vi "CollectionStatus.vi"(8 "error in (no error)":errorcluster, 11 "controller in":refnum<k24>) -> (0 "error out":errorcluster, 1 "PointsCollected":i32, 2 "IsCollecting":bool, 3 "controller out":refnum<k24>, 4 "PointsAllocated":i32, 6 "PointsRetrieved":i32)   [LabVIEW 2016, in "Aerotech VIs.lvlib"]
uses:
  Aerotech VIs.lvlib
  C:/Program Files (x86)/Aerotech/A3200/LabVIEW/2010/Bin/Aerotech.A3200.dll
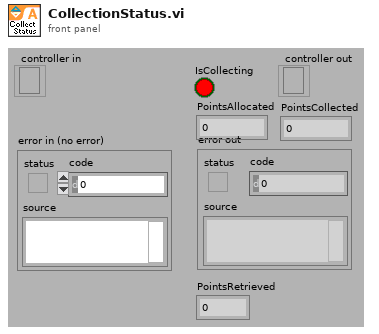
[diagram p1: front panel]
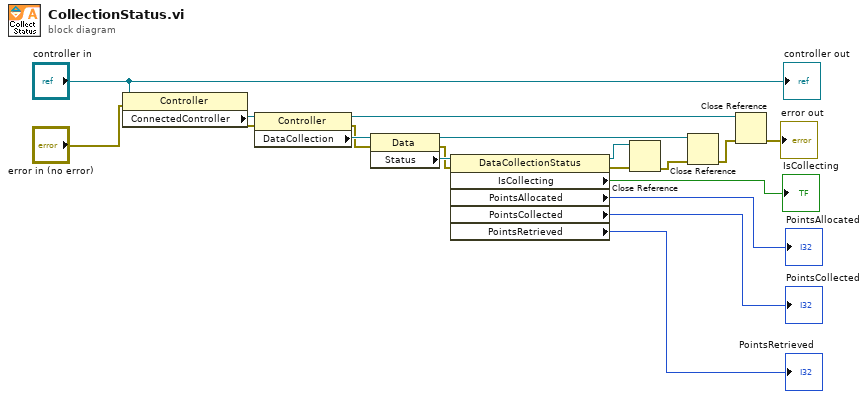
[diagram p0: block diagram]
diagram:
  n1 = property class="Controller"(reference="controller in", error in="error in (no error)") -> (error out=w17:errorcluster, "ConnectedController"=w18:refnum<k24>)  [unwired: 1 out]
  n2 = property class="Controller"(reference=w18, error in=w17) -> (reference out=w10:refnum<k24>, error out=w14:errorcluster, "DataCollection"=w16:refnum<k24>)
  n3 = property class="Data"(reference=w16, error in=w14) -> (reference out=w12:refnum<k24>, error out=w7:errorcluster, "Status"=w8:refnum<k24>)
  n4 = property class="DataCollectionStatus"(reference=w8, error in=w7) -> (reference out=w2:refnum<k24>, error out=w3:errorcluster, "IsCollecting"=→"IsCollecting":bool, "PointsAllocated"=→"PointsAllocated":i32, "PointsCollected"=→"PointsCollected":i32, "PointsRetrieved"=→"PointsRetrieved":i32)
  n5 = Close Reference(reference=w2, error in (no error)=w3) -> (error out=w13:errorcluster)
  n6 = Close Reference(reference=w12, error in (no error)=w13) -> (error out=w11:errorcluster)
  n7 = Close Reference(reference=w10, error in (no error)=w11) -> (error out=→"error out":errorcluster)
  "controller out" <- "controller in"
